vi "GetCurrentStatus.vi"(8 "error in (no error)":errorcluster, 11 "VISA Refnum in":refnum<visa-resource-name>) -> (0 "error out":errorcluster, 2 "status":T1, 3 "VISA resource name out":refnum<visa-resource-name>)   [LabVIEW 2014, in "stepper3D.lvlib"]
uses:
  stepper3D.lvlib
  Enums/CurrentStatus.ctl
  Enums/BoundaryStatus.ctl
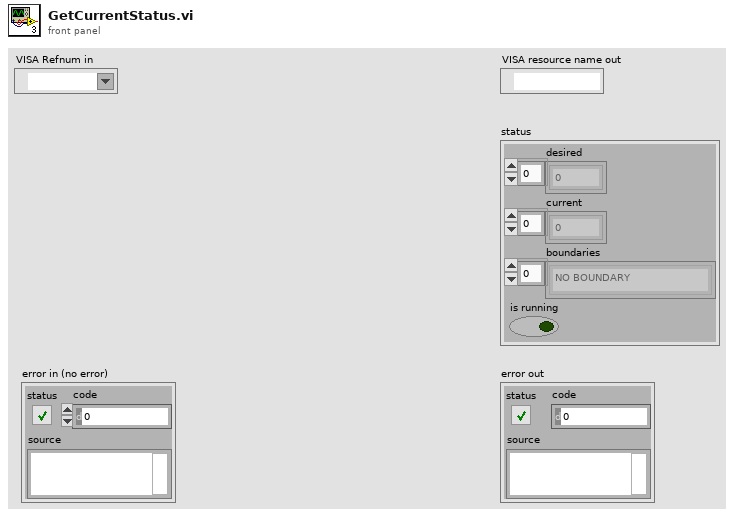
[diagram p1: front panel]
types:
  T1 = typedef "stepper3D.lvlib/CurrentStatus.ctl" = cluster{"desired":dbl[], "current":dbl[], "boundaries":T2[], "is running":bool}
  T2 = typedef "stepper3D.lvlib/BoundaryStatus.ctl" = enum16{"NO BOUNDARY", "OUT OF LEFT", "OUT OF RIGHT"}
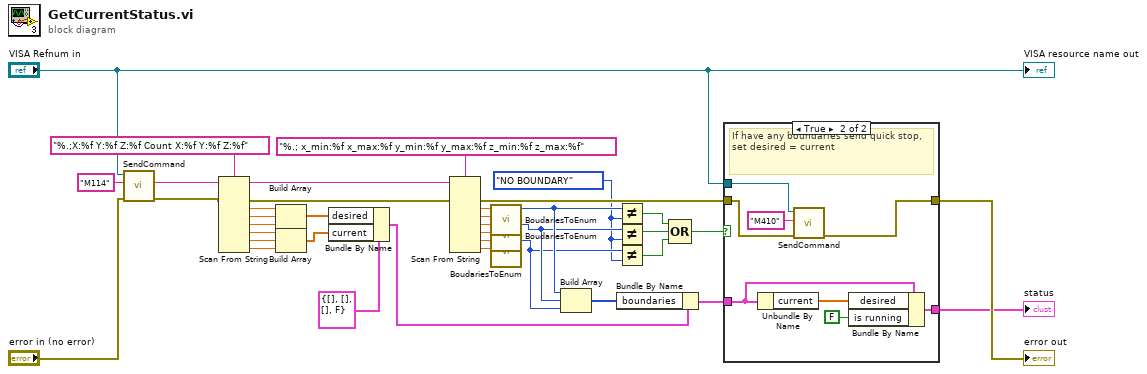
[diagram p0: block diagram]
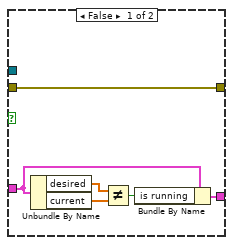
[diagram p2: hidden frame]
diagram:
  w3 = BoundaryStatus."NO BOUNDARY" ("Enum")
  n1 = call "SendCommand.vi"("error in (no error)"="error in (no error)", "command"="M114", "VISA Refnum in"="VISA Refnum in") -> ("error out"=w17:errorcluster, "result"=w36:string)  [unwired: 6 in, 1 out]
  n2 = Scan From String(format string="%.;X:%f Y:%f Z:%f Count X:%f Y:%f Z:%f", input string=w36, error in=w17) -> (remaining string=w25:string, error out=w16:errorcluster, output 1=w35:dbl, output 2=w34:dbl, output 3=w33:dbl, output 4=w32:dbl, output 5=w31:dbl, output 6=w30:dbl)  [unwired: 7 in, 1 out]
  n3 = Build Array(w35, w34, w33) -> (w28:dbl[])
  n4 = Build Array(w32, w31, w30) -> (w26:dbl[])
  n5 = Bundle By Name(cluster=T1 {"desired"=[], "current"=[], "boundaries"=[], "is running"=FALSE} ("result"), "desired"=w28, "current"=w26) -> (w7:T1)
  n6 = Scan From String(format string="%.; x_min:%f x_max:%f y_min:%f y_max:%f z_min:%f z_max:%f", input string=w25, error in=w16) -> (error out=w10:errorcluster, output 1=w23:dbl, output 2=w22:dbl, output 3=w21:dbl, output 4=w20:dbl, output 5=w19:dbl, output 6=w18:dbl)  [unwired: 7 in, 2 out]
  n7 = call "BoudariesToEnum.vi"("max"=w22, "min"=w23) -> ("Enum"=w9:T2)  [unwired: 9 in]
  n8 = call "BoudariesToEnum.vi"("max"=w20, "min"=w21) -> ("Enum"=w8:T2)  [unwired: 9 in]
  n9 = call "BoudariesToEnum.vi"("max"=w18, "min"=w19) -> ("Enum"=w5:T2)  [unwired: 9 in]
  n10 = Build Array(w9, w8, w5) -> (w4:T2[])
  n11 = Not Equal?(x=w9, y=w3) -> (x != y?=w15:bool)
  n12 = Not Equal?(x=w8, y=w3) -> (x != y?=w14:bool)
  n13 = Not Equal?(x=w5, y=w3) -> (x != y?=w13:bool)
  n14 = Bundle By Name(cluster=w7, "boundaries"=w4) -> (w6:T1)
  n15 = Compound Arithmetic op=OR(w15, w14, w13) -> (w12:bool)
  n16 = case shown="True" w12 {
    tunnel: "VISA Refnum in" -> [_ w52]
    tunnel: w10 -> [w44 w50]
    tunnel: w6 -> [w42 w49]
    tunnel: [w43 w47] -> w1
    tunnel: [w44 w46] -> w2
    frame False {
      n17 = Unbundle By Name(w42) -> ("desired"=w41:dbl[], "current"=w40:dbl[])
      n18 = Not Equal?(x=w41, y=w40) -> (x != y?=w39:bool)
      n19 = Bundle By Name(cluster=w42, "is running"=w39) -> (w43:T1)
    }
    frame True {
      # "If have any boundaries send quick stop, set desired = current"
      n20 = Unbundle By Name(w49) -> ("current"=w48:dbl[])
      n21 = call "SendCommand.vi"("error in (no error)"=w50, "command"="M410", "VISA Refnum in"=w52) -> ("error out"=w46:errorcluster)  [unwired: 6 in, 2 out]
      n22 = Bundle By Name(cluster=w49, "desired"=w48, "is running"=FALSE ("IsRunning")) -> (w47:T1)
    }
  }
  "error out" <- w2
  "status" <- w1
  "VISA resource name out" <- "VISA Refnum in"
